vi "integerConversionHelper.vi"(10 "base":i32, 11 "max":i32) -> (2 "base conversion string":string)   [LabVIEW 2014, in "Random JSON API.lvlib"]
uses:
  Random JSON API.lvlib
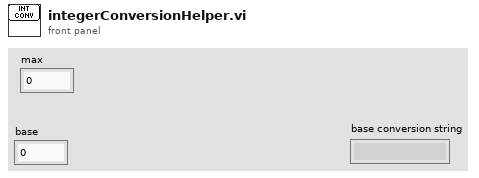
[diagram p1: front panel]
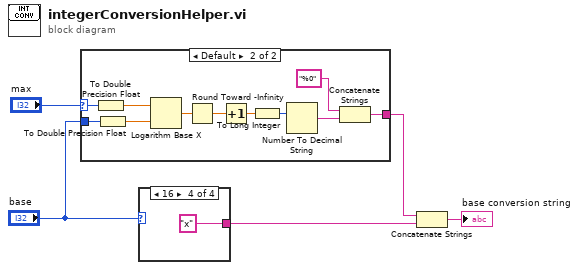
[diagram p0: block diagram]
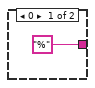
[diagram p2: hidden frame]
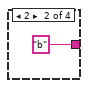
[diagram p4: hidden frame]
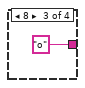
[diagram p5: hidden frame]
diagram:
  n1 = case shown="Default" "max" {
    selector: "max" -> [_ w12]
    tunnel: "base" -> [_ w17]
    tunnel: ["%" ("string") w9] -> w2
    frame 0 {
    }
    frame Default {
      n2 = To Double Precision Float(number=w12) -> (double precision float=w15:dbl)
      n3 = To Double Precision Float(number=w17) -> (double precision float=w16:dbl)
      n4 = Logarithm Base X(1:w16, 2:w15) -> (0:w14:dbl)
      n5 = Round Toward -Infinity(1:w14) -> (0:w13:dbl)
      n6 = Increment(x=w13) -> (x+1=w11:dbl)
      n7 = To Long Integer(number=w11) -> (32bit integer=w10:i32)
      n8 = Number To Decimal String(number=w10) -> (decimal integer string=w8:string)  [unwired: 1 in]
      n9 = Concatenate Strings("%0" ("string"), w8) -> (w9:string)
    }
  }
  n10 = case shown="16" "base" {
    tunnel: [_ "b" ("format string") "o" ("format string") "x" ("format string")] -> w1
    frame Default {
    }
    frame 2 {
    }
    frame 8 {
    }
    frame 16 {
    }
  }
  n11 = Concatenate Strings(w2, w1) -> (→"base conversion string":string)
